vi "UserLogin.vi"() -> ()   [LabVIEW 2021]
uses:
  <vilib>/Utility/file.llb/Write Delimited Spreadsheet (string).vi
  <vilib>/Utility/config.llb/NI_LVConfig.lvlib
panel:
  in  "Tab Control":enum32{"Page 1", "Page 2"}(tab)
  in  "Refresh Button":bool
  in  "Password":string
  in  "User Name:":string
  out "Addition":dbl
  in  "Number 2":dbl
  in  "Number 1":dbl
  in  "stop":bool
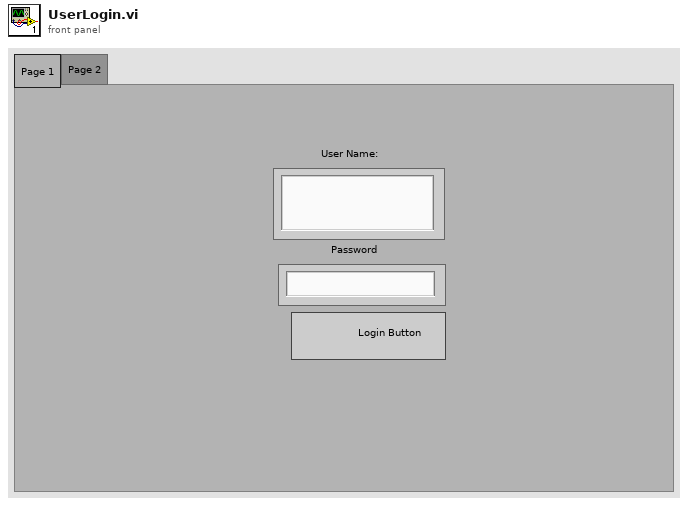
[diagram p1: front panel]
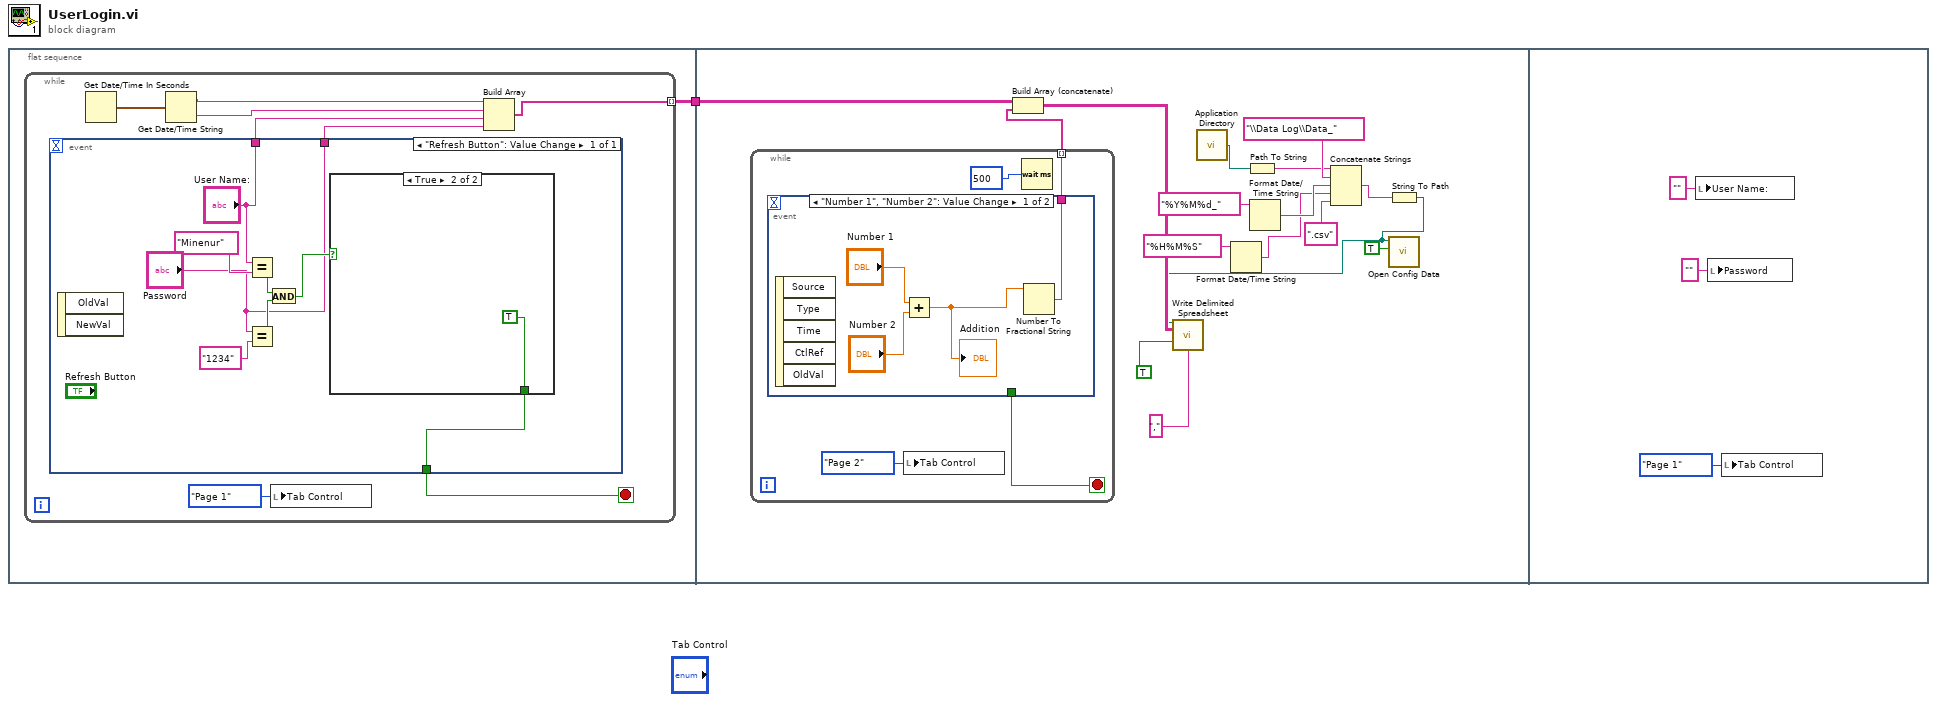
[diagram p0: block diagram]
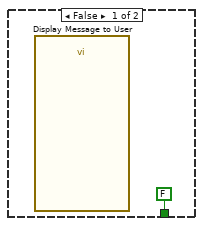
[diagram p2: hidden frame]
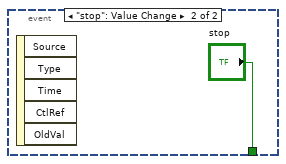
[diagram p3: hidden frame]
diagram:
  n1 = flat-sequence {
    tunnel: [w2] -> w1
    tunnel: w1 -> [w36]
    frame #0 {
      n2 = while {
        tunnel: [w3] -> w2 mode=indexing
        stop <- w10 stop-if-true
        n3 = event shown="[0] \"Refresh Button\": Value Change" {
          selector: _ -> [_]
          dyn-events: _ -> [_]
          timeout: _ -> [_]
          tunnel: [w13] -> w10
          tunnel: ["User Name:"] -> w8
          tunnel: ["Password"] -> w7
          event "Refresh Button": Value Change {
            n4 = event-data() -> ()  [unwired: 1 in, 2 out]
            n5 = Equal?(x="User Name:", y="Minenur" ("Password")) -> (x = y?=w16:bool)
            n6 = Equal?(x="Password", y="1234") -> (x = y?=w15:bool)
            n7 = And(x=w16, y=w15) -> (x .and. y?=w14:bool)
            n8 = case shown="True" w14 {
              tunnel: [FALSE TRUE] -> w13
              frame False {
                n9 = call "Display Message to User"() -> ()  [unwired: 10 in, 2 out]
              }
              frame True {
              }
            }
          }
        }
        n10 = Get Date/Time In Seconds() -> (seconds since 1Jan1904=w6:timestamp)
        n11 = Get Date/Time String(seconds (now)=w6) -> (date string=w5:string, time string=w4:string)  [unwired: 2 in]
        n12 = local write "Tab Control"(enum32{"Page 1", "Page 2"}."Page 1" ("Tab Control")) -> ()
        n13 = Build Array(w5, w4, w8, w7) -> (w3:string[])
      }
    }
    frame #1 {
      n14 = while {
        tunnel: [w37] -> w35 mode=indexing
        stop <- w38 stop-if-true
        n15 = event shown="[0] \"Number 1\", \"Number 2\": Value Change" {
          selector: _ -> [_ _]
          dyn-events: _ -> [_ _]
          timeout: _ -> [_ _]
          tunnel: [_ "stop"] -> w38
          tunnel: [w41 _] -> w37
          event "Number 1", "Number 2": Value Change {
            n16 = event-data() -> ()  [unwired: 1 in, 5 out]
            n17 = Add(x="Number 1", y="Number 2") -> (x+y=w42:dbl)
            "Addition" <- w42
            n18 = Number To Fractional String(number=w42) -> (F-format string=w41:string)  [unwired: 3 in]
          }
          event "stop": Value Change {
            n19 = event-data() -> ()  [unwired: 1 in, 5 out]
          }
        }
        n20 = local write "Tab Control"(enum32{"Page 1", "Page 2"}."Page 2" ("Tab Control")) -> ()
        n21 = Wait (ms)(milliseconds to wait=u32 500 ("millisecond timer value")) -> ()  [unwired: 1 out]
      }
      n22 = Build Array (concatenate)(w36, w35) -> (w34:string[][])
      n23 = call <vilib>:"Application Directory.vi"() -> ("Application Directory"=w31:path)
      n24 = Format Date/Time String(time format string (%c)="%H%M%S") -> (date/time string=w21:string)  [unwired: 2 in]
      n25 = Path To String(path=w31) -> (string=w25:string)
      n26 = Format Date/Time String(time format string (%c)="%Y%M%d_") -> (date/time string=w22:string)  [unwired: 2 in]
      n27 = Concatenate Strings(w25, "\\Data Log\\Data_" ("string"), w22, w21, ".csv" ("element")) -> (w29:string)
      n28 = String To Path(string=w29) -> (path=w28:path)
      n29 = call-poly <vilib>:"Write Delimited Spreadsheet.vi"("file path (dialog if empty)"=w28, "2D data"=w34, "append to file? (new file:F)"=TRUE, "delimiter (\\t)"="," ("delimiter (\\t)")) -> ()  [unwired: 10 in, 2 out]
      n30 = call <vilib>:"Open Config Data.vi"("create file if necessary (T)"=TRUE, "configuration file path"=w28) -> ()  [unwired: 7 in, 3 out]
    }
    frame #2 {
      n31 = local write "User Name:"("" ("User Name:")) -> ()
      n32 = local write "Password"("" ("Password")) -> ()
      n33 = local write "Tab Control"(enum32{"Page 1", "Page 2"}."Page 1" ("Tab Control")) -> ()
    }
  }
